vi "Complementary Filter -DMP.vi"() -> ()   [LabVIEW 2014]
uses:
  <userlib>/UCSD Robotics Lab/Robotics-Cape/LV/libroboticscape.lvlib
panel:
  out "Error":dbl format="%#_2f"
  out "Complementary Filter Output":T1
  out "Waveform Chart":T2(graph)
  in  "Filter Time Constant":dbl=1.0 format="%#_13g"
  out "State":T3(ring)
  out "Timing Block":T4 {"Actual Hz" format="%#_3g"; "Dt" format="%#_4g"; "Average Hz" format="%#_4g"}
  in  "Input Prior to Start":T5={"orientation"=112, "IMU_sample_rate "=200, "dmp_interrupt_priority"=98} {"dmp_interrupt_priority" min=1 max=99 step=1; "IMU_sample_rate" min=4 max=200; "orientation" items=["ORIENTATION_Z_UP"=136, "ORIENTATION_Z_DOWN"=396, "ORIENTATION_X_UP"=14, "ORIENTATION_X_DOWN"=266, "ORIENTATION_Y_UP"=112, "ORIENTATION_Y_DOWN"=336, "ORIENTATION_X_FORWARD"=133, "ORIENTATION_X_BACK"=161]}
  in  "stop":bool
  # "Always stop the VI using the rectangular STOP button below, never with the round stopsign (Abort)"
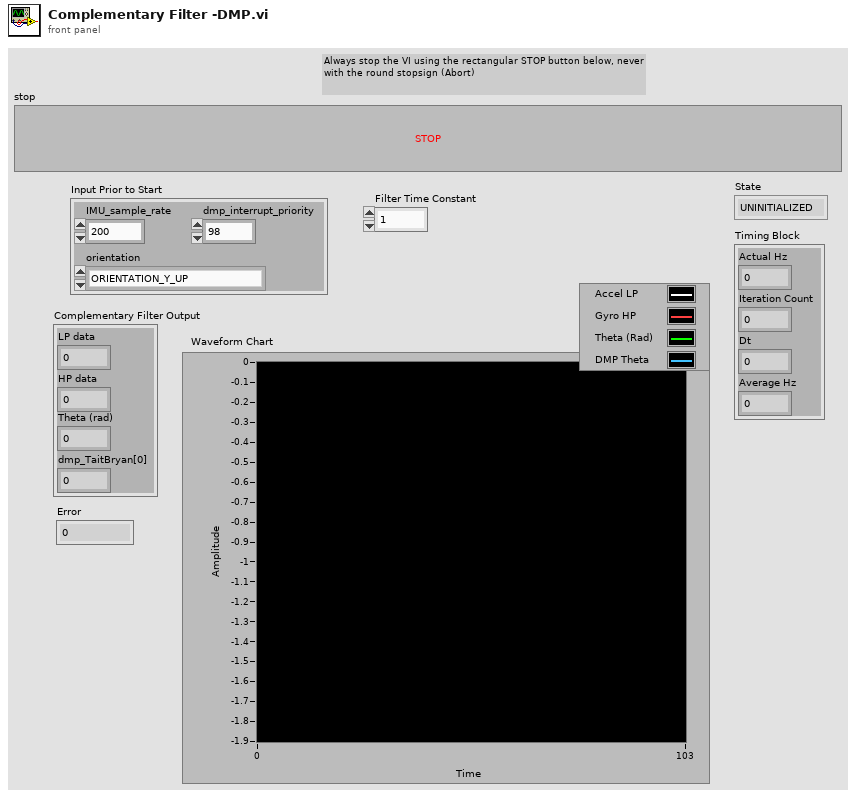
[diagram p1: front panel]
types:
  T1 = cluster{"LP data":dbl, "HP data":dbl, "Theta (rad)":dbl, "dmp_TaitBryan[0]":sgl}
  T2 = cluster{"LP data":dbl, "HP data":dbl, dbl, "dmp_TaitBryan[0]":sgl}
  T3 = enum16{"UNINITIALIZED", "RUNNING", "PAUSED", "EXITING"}
  T4 = cluster{"Actual Hz":dbl, "Iteration Count":dbl, "Dt":dbl, "Average Hz":dbl}
  T5 = cluster{"orientation":u32, "IMU_sample_rate ":i32, "dmp_interrupt_priority":i32}
  T6 = cluster{"accel[0]":sgl, "accel[1]":sgl, "accel[2]":sgl, "gyro[0]":sgl, "gyro[1]":sgl, "gyro[2]":sgl, "mag[0]":sgl, "mag[1]":sgl, "mag[2]":sgl, "temp":sgl, "raw_gyro[0]":i16, "raw_gyro[1]":i16, "raw_gyro[2]":i16, "raw_accel[0]":i16, "raw_accel[1]":i16, "raw_accel[2]":i16, "accel_to_ms2":sgl, "gyro_to_degs":sgl, "dmp_quat[0]":sgl, "dmp_quat[1]":sgl, "dmp_quat[2]":sgl, "dmp_quat[3]":sgl, "dmp_TaitBryan[0]":sgl, "dmp_TaitBryan[1]":sgl, "dmp_TaitBryan[2]":sgl, "fused_quat[0]":sgl, "fused_quat[1]":sgl, "fused_quat[2]":sgl, "fused_quat[3]":sgl, "fused_TaitBryan[0]":sgl, "fused_TaitBryan[1]":sgl, "fused_TaitBryan[2]":sgl, "compass_heading":sgl, "compass_heading_raw":sgl}
  T7 = enum16{"UNINITIALIZED", "RUNING", "PAUSED", "EXITING"}
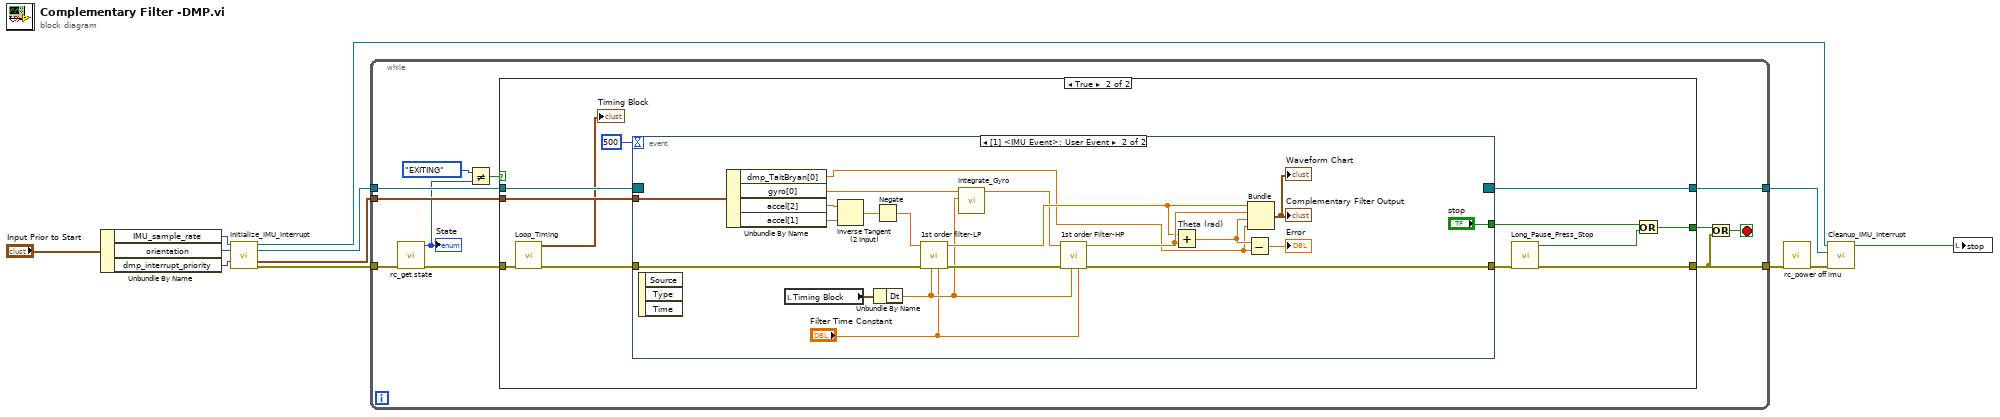
[diagram p0: block diagram]
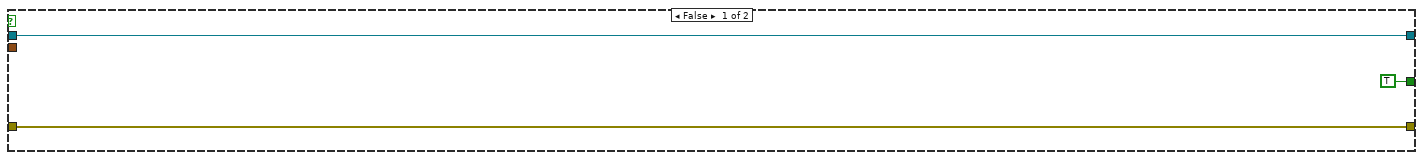
[diagram p2: hidden frame]
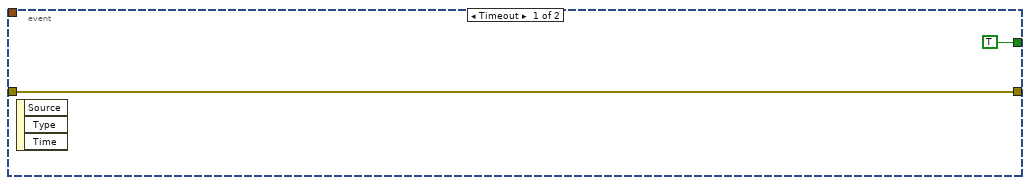
[diagram p3: hidden frame]
diagram:
  n1 = Unbundle By Name("Input Prior to Start") -> ("IMU_sample_rate"=w5:i32, "orientation"=w4:u32, "dmp_interrupt_priority"=w3:i32)
  n2 = call "Initialize_IMU_Interrupt.vi"("dmp_sample_rate"=w5, "orientation"=w4, "dmp_interrupt_priority"=w3) -> ("IMU Event"=w10:refnum<user-event>, "Event Registration Refnum"=w12:refnum<event-registration>, "IMU Data"=w8:T6, "error out"=w7:errorcluster)  [unwired: 9 in]
  n3 = while {
    tunnel: w7 -> [w18]
    tunnel: [w23] -> w9
    tunnel: [w21] -> w2
    tunnel: w12 -> [w22]
    tunnel: w8 -> [w19]
    stop <- w20 stop-if-true
    n4 = call <userlib>:"rc_get state.vi"("error in (no error)"=w18) -> ("error out"=w17:errorcluster, "function return"=w13:u32)  [unwired: 9 in]
    "State" <- w13
    n5 = Not Equal?(x=T7."EXITING" ("State 2"), y=w13) -> (x != y?=w15:bool)
    n6 = case shown="True" w15 {
      tunnel: [w25 w38] -> w23
      tunnel: w22 -> [w25 w36]
      tunnel: [w26 w32] -> w21
      tunnel: w19 -> [_ w35]
      tunnel: w17 -> [w26 w34]
      tunnel: [TRUE ("stop") w30] -> w14
      frame False {
      }
      frame True {
        n7 = call "Loop_Timing.vi"("error in"=w34) -> ("error out"=w33:errorcluster, "Timing Block"=→"Timing Block":T4)  [unwired: 9 in]
        n8 = event shown="[1] <IMU Event>: User Event" {
          selector: w36 -> [_ _]
          dyn-events: [_ _] -> w38
          timeout: 500 -> [_ _]
          tunnel: w33 -> [w40 w56]
          tunnel: [w40 w54] -> w28
          tunnel: w35 -> [_ w59]
          tunnel: [TRUE ("stop") "stop"] -> w27
          event Timeout {
            n9 = event-data() -> ()  [unwired: 1 in, 3 out]
          }
          event User Event {
            n10 = event-data() -> ()  [unwired: 1 in, 3 out]
            n11 = Unbundle By Name(w59) -> ("dmp_TaitBryan[0]"=w42:sgl, "gyro[0]"=w43:sgl, "accel[2]"=w44:sgl, "accel[1]"=w45:sgl)
            n12 = local read "Timing Block"() -> (w57:T4)
            n13 = Inverse Tangent (2 Input)(1:w45, 2:w44) -> (0:w58:sgl)
            n14 = Unbundle By Name(w57) -> ("Dt"=w47:dbl)
            n15 = Negate(x=w58) -> (-x=w49:sgl)
            n16 = call "1st order filter-LP.vi"("Filter Time Constant"="Filter Time Constant", "Dt"=w47, "error in"=w56, "Data in"=w49) -> ("error out"=w55:errorcluster, "LP data"=w50:dbl)  [unwired: 6 in]
            n17 = call "Integrate_Gyro.vi"("Dt"=w47, "gyro[0]"=w43) -> ("Integrated Gyro"=w48:dbl)  [unwired: 9 in]
            n18 = call "1st order Filter-HP.vi"("Filter Time Constant"="Filter Time Constant", "Dt"=w47, "error in"=w55, "Data in"=w48) -> ("error out"=w54:errorcluster, "HP data"=w51:dbl)  [unwired: 6 in]
            n19 = Add "Theta (rad)"(x=w50, y=w51) -> (x+y=w52:dbl)
            n20 = Subtract(x=w52, y=w42) -> (x-y=→"Error":dbl)
            n21 = Bundle("LP data"=w50, "HP data"=w51, w52, "dmp_TaitBryan[0]"=w42) -> (→"Waveform Chart" →"Complementary Filter Output":T2)  [unwired: 1 in]
          }
        }
        n22 = call "Long_Pause_Press_Stop.vi"("error in (no error)"=w28) -> ("error out"=w32:errorcluster, "Stop"=w31:bool)  [unwired: 9 in]
        n23 = Or(x=w27, y=w31) -> (x .or. y?=w30:bool)
      }
    }
    n24 = Or(x=w14, y=w21) -> (x .or. y?=w20:bool)
  }
  n25 = call <userlib>:"rc_power off imu.vi"("error in (no error)"=w2) -> ("error out"=w1:errorcluster)  [unwired: 9 in, 1 out]
  n26 = call "Cleanup_IMU_Interrupt.vi"("error in (no error)"=w1, "Event Registration Refnum 2"=w9, "IMU Event"=w10) -> ("Stop Local Variabl"=w11:bool)  [unwired: 6 in]
  n27 = local write "stop"(w11) -> ()
